vi "Check Channel.vi"(7 "Peripheral":T7, 8 "Error In":errorcluster, 10 "Channels":u8[](array[numeric]), 11 "LINX Resource":T1) -> (0 "Error Out":errorcluster, 2 "Channels":u8[](array[numeric]), 3 "LINX Resource":T1)   [LabVIEW 2013, in "LVH-LINX.lvlib"]
doc: "Generate an error if the specified channel does not exist on the current device."
uses:
  <vilib>/LabVIEW Hacker/LINX/LVH-LINX.lvlib
  <vilib>/LabVIEW Hacker/LINX/Private/Type Defs/Peripheral.ctl
  <vilib>/LabVIEW Hacker/LINX/Private/Type Defs/LINX Ref.ctl
  <vilib>/LabVIEW Hacker/LINX/Private/Type Defs/Platform.ctl
  <vilib>/LabVIEW Hacker/LINX/Private/Type Defs/Interface.ctl
  <vilib>/LabVIEW Hacker/LINX/Private/Device/Type Defs/LINX Device Config.ctl
  <vilib>/LabVIEW Hacker/LINX/Private/Device/Type Defs/TCP Config.ctl
  <vilib>/LabVIEW Hacker/LINX/Private/Type Defs/Device Family.ctl
  <vilib>/LabVIEW Hacker/LINX/Private/Type Defs/Error Type.ctl
  <vilib>/LabVIEW Hacker/LINX/Private/Device/Device.lvlib
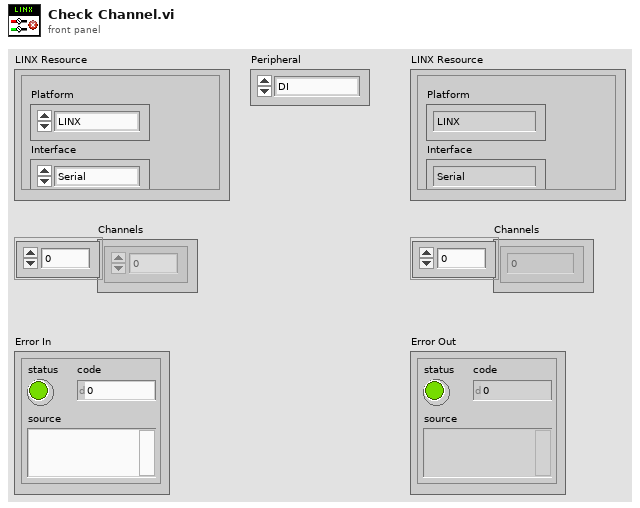
[diagram p1: front panel]
types:
  T1 = typedef "LVH-LINX.lvlib/LINX Ref.ctl" = cluster{"Platform":T2, "Interface":T3, "LINX Device Config":T4}
  T2 = typedef "LVH-LINX.lvlib/Platform.ctl" = enum16{"LINX", "myRIO"}
  T3 = typedef "LVH-LINX.lvlib/Interface.ctl" = enum16{"Serial", "TCP"}
  T4 = typedef "LVH-LINX.lvlib/Device.lvlib/LINX Device Config.ctl" = cluster{"Interface":T3, "COM Port":refnum<visa-resource-name>, "TCP Configuration":T5, "Device Family":T6, "Device ID":u8, "Device Name":string, "TCP Ref":refnum<k5>}
  T5 = typedef "LVH-LINX.lvlib/Device.lvlib/TCP Config.ctl" = cluster{"IP Address":string, "Port":u16}
  T6 = typedef "LVH-LINX.lvlib/Device Family.ctl" = enum8{"National Instruments", "Digilent", "Arduino"}
  T7 = typedef "LVH-LINX.lvlib/Peripheral.ctl" = enum8{"DI", "DO", "AI", "AO", "PWM", "QE", "UART", "I2C", "SPI", "CAN"}
  T8 = typedef "LVH-LINX.lvlib/Generic Device.ctl" = cluster{"DI Channels":u8[], "DO Channels":u8[], "AI":u8[], "AO":u8[], "PWM":u8[], "QE":u8[], "UART":u8[], "I2C 2":u8[], "SPI":u8[], "CAN":u8[], "AI Ref (V)":dbl, "Firmware Program Interfaces":enum16{"N/A", "Serial / USB", "USB", "TCP"}[], "Firmware Versions":T9[], "Name":string, "AO Resolution (Bits)":u8, "AO Ref (V)":dbl}
  T9 = typedef "LVH-LINX.lvlib/Firmware Version.ctl" = cluster{"Name":string, "Relative Path":string, "Firmware Interface":T10}
  T10 = typedef "LVH-LINX.lvlib/Firmware Interface.ctl" = enum32{"Serial ", "Ethernet", "WIFI"}
  T11 = typedef "LVH-LINX.lvlib/Error Type.ctl" = enum16{"Unknown", "Timeout", "Corrupt Return Packet", "Unable To Connect", "Command Not Supported", "Channel DNE", "Invalid COM Config"}
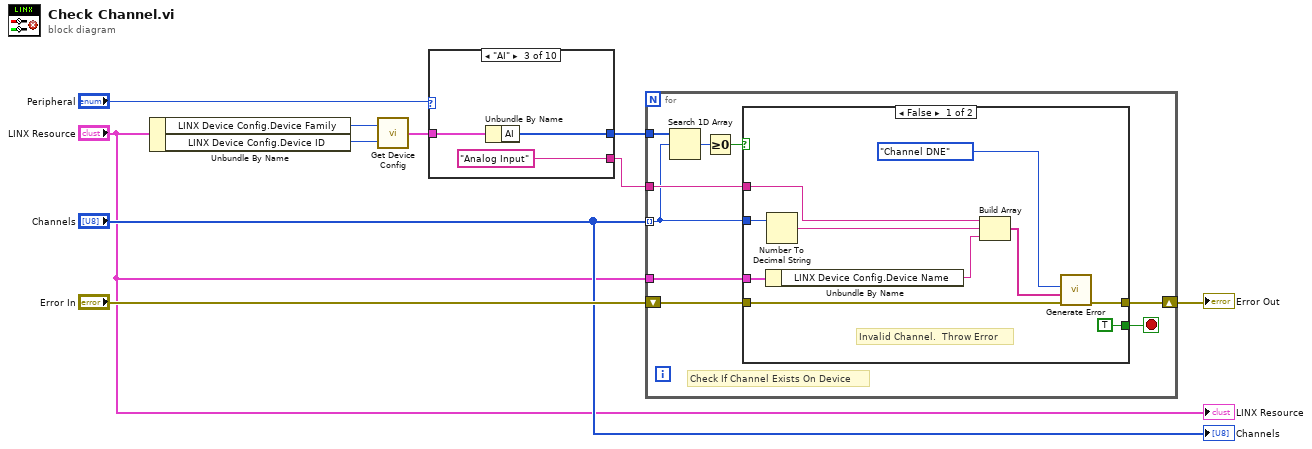
[diagram p0: block diagram]
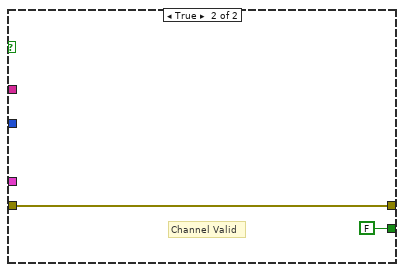
[diagram p2: hidden frame]
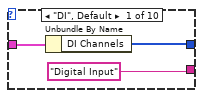
[diagram p3: hidden frame]
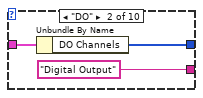
[diagram p4: hidden frame]
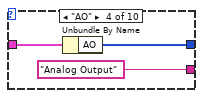
[diagram p5: hidden frame]
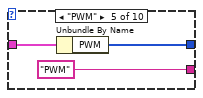
[diagram p6: hidden frame]
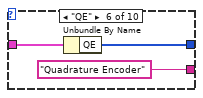
[diagram p7: hidden frame]
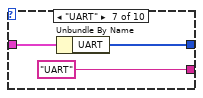
[diagram p8: hidden frame]
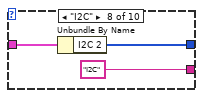
[diagram p9: hidden frame]
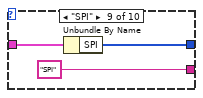
[diagram p10: hidden frame]
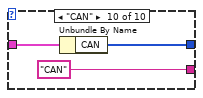
[diagram p11: hidden frame]
diagram:
  n1 = Unbundle By Name("LINX Resource") -> ("LINX Device Config.Device Family"=w2:T6, "LINX Device Config.Device ID"=w1:u8)
  n2 = call <vilib>:"Get Device Config.vi"("Device ID"=w1, "Device Family"=w2) -> ("Device Config"=w4:T8)
  n3 = case shown="\"AI\"" "Peripheral" {
    tunnel: w4 -> [w13 w16 w19 w22 w25 w28 w31 w34 w37 w40]
    tunnel: [w12 w15 w18 w21 w24 w27 w30 w33 w36 w39] -> w9
    tunnel: ["Digital Input" "Digital Output" "Analog Input" "Analog Output" "PWM" "Quadrature Encoder" "UART" "I2C" "SPI" "CAN"] -> w7
    frame "DI", Default {
      n4 = Unbundle By Name(w13) -> ("DI Channels"=w12:u8[])
    }
    frame "DO" {
      n5 = Unbundle By Name(w16) -> ("DO Channels"=w15:u8[])
    }
    frame "AI" {
      n6 = Unbundle By Name(w19) -> ("AI"=w18:u8[])
    }
    frame "AO" {
      n7 = Unbundle By Name(w22) -> ("AO"=w21:u8[])
    }
    frame "PWM" {
      n8 = Unbundle By Name(w25) -> ("PWM"=w24:u8[])
    }
    frame "QE" {
      n9 = Unbundle By Name(w28) -> ("QE"=w27:u8[])
    }
    frame "UART" {
      n10 = Unbundle By Name(w31) -> ("UART"=w30:u8[])
    }
    frame "I2C" {
      n11 = Unbundle By Name(w34) -> ("I2C 2"=w33:u8[])
    }
    frame "SPI" {
      n12 = Unbundle By Name(w37) -> ("SPI"=w36:u8[])
    }
    frame "CAN" {
      n13 = Unbundle By Name(w40) -> ("CAN"=w39:u8[])
    }
  }
  n14 = for {
    shift-right: [w47] -> w6
    shift-left: "Error In" -> [w46]
    tunnel: "Channels" -> [w42] mode=indexing
    tunnel: w9 -> [w44]
    tunnel: w7 -> [w43]
    tunnel: "LINX Resource" -> [w41]
    stop <- w45 stop-if-true
    # "Check If Channel Exists On Device"
    n15 = Search 1D Array(1D array=w44, element=w42) -> (index of element=w49:i32)  [unwired: 1 in]
    n16 = Greater Or Equal To 0?(x=w49) -> (x >= 0?=w48:bool)
    n17 = case shown="False" w48 {
      tunnel: [w57 w61] -> w47
      tunnel: w46 -> [w58 w61]
      tunnel: [TRUE FALSE] -> w45
      tunnel: w43 -> [w55 _]
      tunnel: w42 -> [w56 _]
      tunnel: w41 -> [w52 _]
      frame False {
        # "Invalid Channel.  Throw Error"
        n18 = Unbundle By Name(w52) -> ("LINX Device Config.Device Name"=w53:string)
        n19 = Number To Decimal String(number=w56) -> (decimal integer string=w54:string)  [unwired: 1 in]
        n20 = Build Array(w55, w54, w53) -> (w50:string[])
        n21 = call <vilib>:"Generate Error.vi"("Error In"=w58, "Arguments"=w50, "Error Type"=Error_Type."Channel DNE") -> ("Error Out"=w57:errorcluster)  [unwired: 7 in, 1 out]
      }
      frame True {
        # "Channel Valid"
      }
    }
  }
  "Error Out" <- w6
  "Channels" <- "Channels"
  "LINX Resource" <- "LINX Resource"
